vi "mod_Resample profile to requested sampling rate.vi"(0 "doppler filter output":cdb[](array[numeric]), 5 "interpolating filter":dbl[](array[numeric]) format="%.2f", 7 "profile length (samples)":i32=1000, 9 "interpolation factor":i32=1, 11 "error in (no error)":errorcluster, 13 "reset? (T)":bool=TRUE) -> (4 "fading profile":cdb[](array[numeric]), 15 "error out":errorcluster)   [LabVIEW 2020, in "niDMT.lvlib"]
uses:
  <vilib>/addons/Modulation/niDMT.lvlib
  <vilib>/addons/Modulation/Analog/support/mod_Interpolating FIR.vi
  <vilib>/Analysis/3filter.llb/IIR Filter with I.C..vi
  <vilib>/Analysis/3filter.llb/IIR Filter with I.C. (DBL).vi
  <vilib>/addons/Modulation/niAMT.lvlib
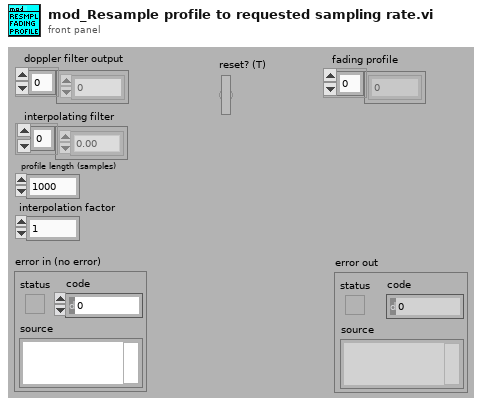
[diagram p1: front panel]
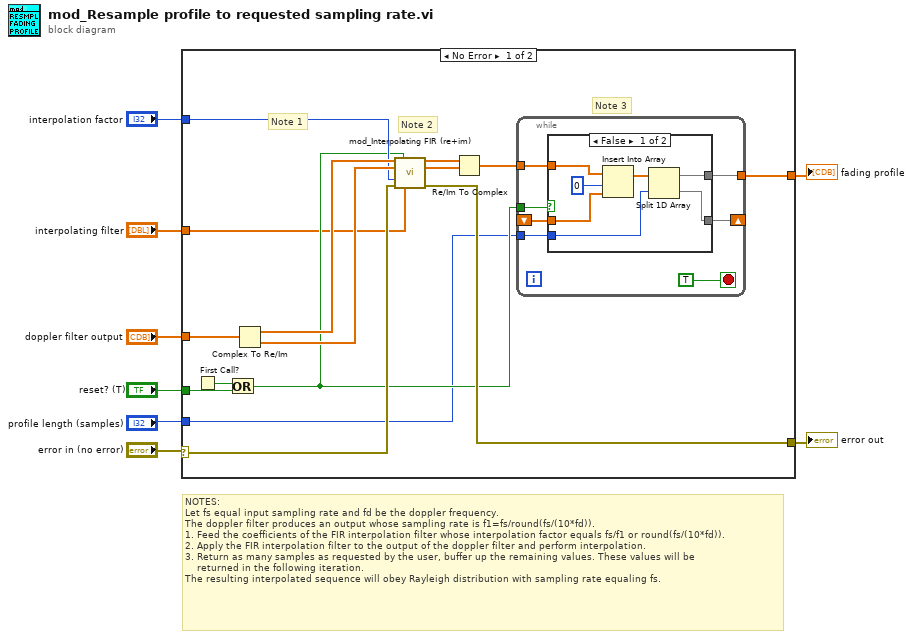
[diagram p0: block diagram]
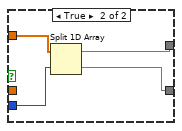
[diagram p2: hidden frame]
diagram:
  # "NOTES:\nLet fs equal input sampling rate and fd be the doppler frequency.\nThe doppler filter produces an output whose sampling rate is f1=fs/round(fs/(10*fd)).\n1. Feed the coefficients of the FIR interpolation filter whose interpolation factor equals fs/f1 or round(fs/(10*fd)).\n2. Apply the FIR interpolation filter to the output of the doppler filter and perform interpolation.\n3. Return as many samples as requested by the user, buffer up the remaining values. These values will be \n    returned in the following iteration.\nThe resulting interpolated sequence will obey Rayleigh distribution with sampling rate equaling fs."
  n1 = case shown="No Error" "error in (no error)" {
    selector: "error in (no error)" -> [w17 w42]
    tunnel: "interpolation factor" -> [w18 _]
    tunnel: "reset? (T)" -> [w23 _]
    tunnel: "profile length (samples)" -> [w11 _]
    tunnel: "doppler filter output" -> [w21 _]
    tunnel: [w14 w42] -> w3
    tunnel: [w10 _] -> w2
    tunnel: "interpolating filter" -> [w9 _]
    frame No Error {
      # "Note 3"
      # "Note 2"
      # "Note 1"
      n2 = First Call?() -> (First Call?: T/F=w22:bool)
      n3 = Or(x=w22, y=w23) -> (x .or. y?=w13:bool)
      n4 = Complex To Re/Im(x + iy=w21) -> (x=w20:dbl[], y=w19:dbl[])
      n5 = call <vilib>:"mod_Interpolating FIR (re+im).vi"("Real in"=w20, "Reset"=w13, "Im in"=w19, "interpolation"=w18, "error in (no error)"=w17, "taps"=w9) -> ("Real out"=w16:dbl[], "im out"=w15:dbl[], "error out"=w14:errorcluster)  [unwired: 7 out]
      n6 = Re/Im To Complex(1:w15, 2:w16) -> (0:w12:cdb[])
      n7 = while {
        tunnel: w13 -> [w29]
        tunnel: w12 -> [w28]
        tunnel: w11 -> [w27]
        shift-right: [w26] -> _
        shift-left: _ -> [w25]
        tunnel: [w24] -> w10
        stop <- TRUE stop-if-true
        n8 = case shown="False" w29 {
          tunnel: w28 -> [w37 w41]
          tunnel: w27 -> [w33 w40]
          tunnel: [w32 w39] -> w26
          tunnel: w25 -> [w35 _]
          tunnel: [w31 w38] -> w24
          frame False {
            n9 = Insert Into Array(array=w37, index=0, new element=w35) -> (w34:cdb[])
            n10 = Split 1D Array(array=w34, index=w33) -> (first subarray=w31:cdb[], second subarray=w32:cdb[])
          }
          frame True {
            n11 = Split 1D Array(array=w41, index=w40) -> (first subarray=w38:cdb[], second subarray=w39:cdb[])
          }
        }
      }
    }
    frame Error {
    }
  }
  "error out" <- w3
  "fading profile" <- w2
